vi "数组创建.vi"() -> ()   [LabVIEW 2018]
panel:
  in  "数组":dbl[][](array[numeric])
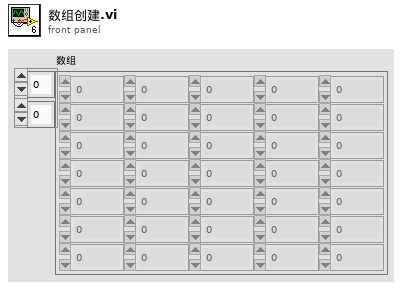
[diagram p1: front panel]
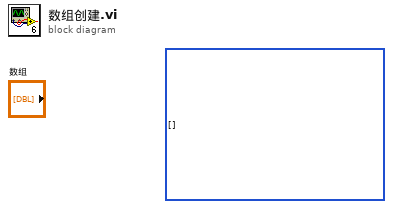
[diagram p0: block diagram]
diagram:
  (unwired) i32[][] []
